vi "test_ClientFGV_RecreateClientErrors_ClientNotCreated.vi"(8 "error in":errorcluster) -> (0 "error out":errorcluster, 2 "result":string, 3 "pass":bool)   [LabVIEW 2020, in "MeasurementServerTests.lvlib" / "Discovery Tests.lvlib"]
uses:
  Discovery Tests.lvlib
  Runtime/APIs/Discovery V1/TypeDefs/gRPC Client Cache FGV Action.ctl
  Runtime/APIs/Discovery V1/Plug-In SDK Discovery V1 API.lvlib
  Fake Client Id Generator Action.ctl
  MeasurementServerTests.lvlib
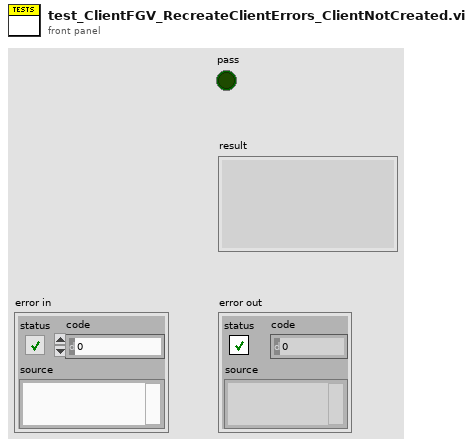
[diagram p1: front panel]
types:
  T1 = typedef "MeasurementServerTests.lvlib/Discovery Tests.lvlib/Fake Client Id Generator Action.ctl" = enum16{"Generate New Id", "Reset", "Error on Next Call"}
  T2 = typedef "Plug-In SDK Discovery V1 API.lvlib/gRPC Client Cache FGV Action.ctl" = enum16{"Get Client", "Recreate Client", "Destroy Client", "Update ClusterId"}
  T3 = typedef "grpc-lvsupport-release.lvlib/grpcId.ctl" = u64
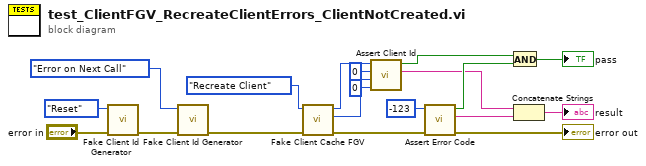
[diagram p0: block diagram]
diagram:
  n1 = call "Fake Client Id Generator.vi"("error in"="error in", "action"=Fake_Client_Id_Generator_Action."Reset") -> ("error out"=w14:errorcluster)  [unwired: 8 in, 1 out]
  n2 = call "Fake Client Id Generator.vi"("error in"=w14, "action"=Fake_Client_Id_Generator_Action."Error on Next Call") -> ("error out"=w15:errorcluster)  [unwired: 8 in, 1 out]
  n3 = call "Fake Client Cache FGV.vi"("error in"=w15, "action"=gRPC_Client_Cache_FGV_Action."Recreate Client") -> ("error out"=w13:errorcluster, "unique id out"=w9:u64, "grpc client id"=w10:T3)  [unwired: 7 in]
  n4 = call "Assert Client Id.vi"("expected unique id"=u64 0, "actual unique id"=w9, "expected client id"=u64 0, "actual client id"=w10) -> ("result"=w3:string, "pass"=w6:bool)  [unwired: 6 in]
  n5 = call "Assert Error Code.vi"("error in"=w13, "expected error code"=-123) -> ("error out"=→"error out":errorcluster, "details"=w2:string, "error code match?"=w5:bool)  [unwired: 7 in]
  n6 = And(x=w6, y=w5) -> (x .and. y?=→"pass":bool)
  n7 = Concatenate Strings(w3, w2) -> (→"result":string)
